vi "drive_globals.vi"() -> ()   [LabVIEW 2020]
panel:
  out "Drive Target BR":dbl
  out "Azimuth Target BR":dbl
  out "Drive Target BL":dbl
  out "Azimuth Target BL":dbl
  out "Drive Target FL":dbl
  out "Azimuth Target FL":dbl
  out "Azimuth Target FR":dbl
  out "Drive Target FR":dbl
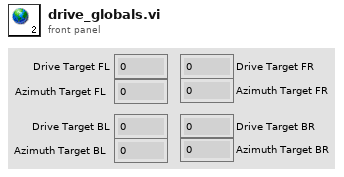
[diagram p1: front panel]
diagram:
